vi "VBAI_MeasurementReader.vi"() -> ()   [LabVIEW 2014]
uses:
  g_Stop.vi
  g_VBAIMeasurements.vi
panel:
  in  "stop":bool
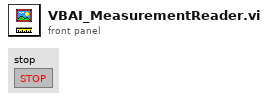
[diagram p1: front panel]
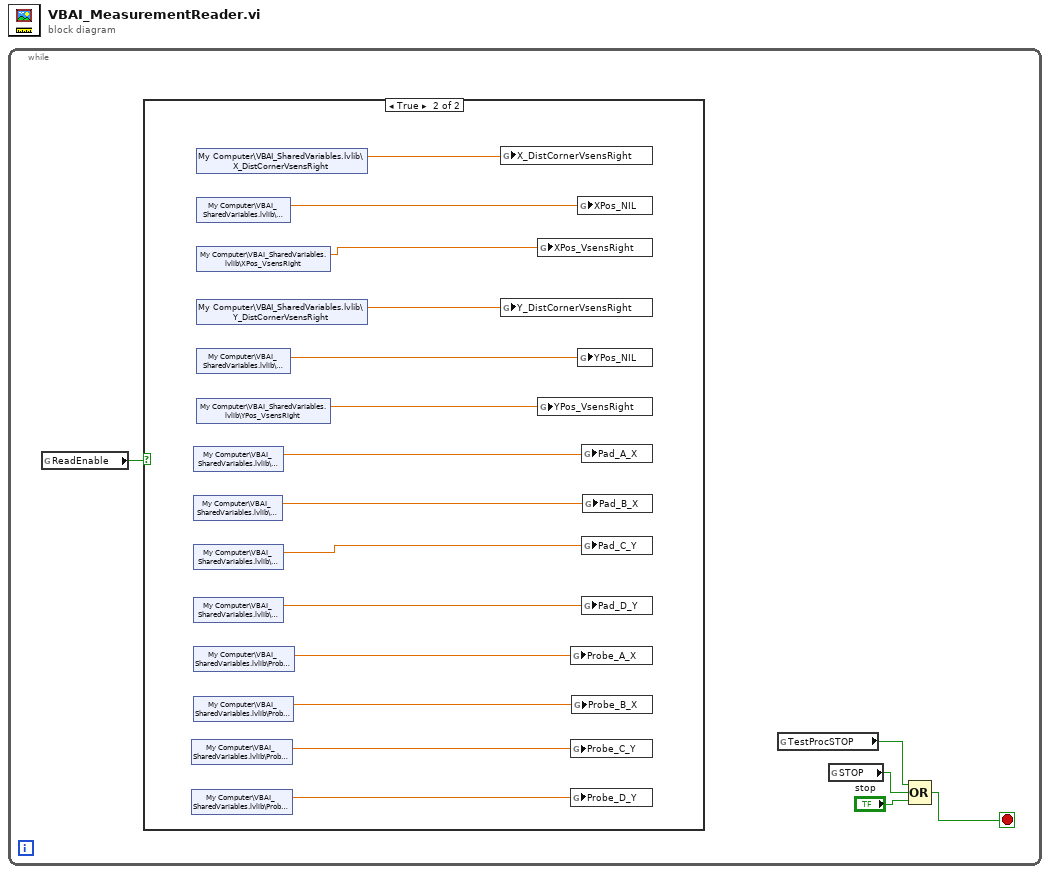
[diagram p0: block diagram]
diagram:
  n1 = while {
    stop <- w4 stop-if-true
    n2 = global read "g_VBAIMeasurements.vi" "ReadEnable"() -> (w1:bool)
    n3 = case shown="True" w1 {
      frame False {
      }
      frame True {
        n4 = shared-variable "My Computer\\VBAI_SharedVariables.lvlib\\Probe_C_Y"() -> (w7:dbl)  [unwired: 1 in, 1 out]
        n5 = shared-variable "My Computer\\VBAI_SharedVariables.lvlib\\Probe_D_Y"() -> (w6:dbl)  [unwired: 1 in, 1 out]
        n6 = shared-variable "My Computer\\VBAI_SharedVariables.lvlib\\Pad_A_X"() -> (w8:dbl)  [unwired: 1 in, 1 out]
        n7 = shared-variable "My Computer\\VBAI_SharedVariables.lvlib\\Pad_B_X"() -> (w9:dbl)  [unwired: 1 in, 1 out]
        n8 = shared-variable "My Computer\\VBAI_SharedVariables.lvlib\\Pad_C_Y"() -> (w10:dbl)  [unwired: 1 in, 1 out]
        n9 = shared-variable "My Computer\\VBAI_SharedVariables.lvlib\\Pad_D_Y"() -> (w11:dbl)  [unwired: 1 in, 1 out]
        n10 = shared-variable "My Computer\\VBAI_SharedVariables.lvlib\\Probe_A_X"() -> (w12:dbl)  [unwired: 1 in, 1 out]
        n11 = shared-variable "My Computer\\VBAI_SharedVariables.lvlib\\Probe_B_X"() -> (w13:dbl)  [unwired: 1 in, 1 out]
        n12 = shared-variable "My Computer\\VBAI_SharedVariables.lvlib\\X_DistCornerVsensRight"() -> (w19:dbl)  [unwired: 1 in, 1 out]
        n13 = shared-variable "My Computer\\VBAI_SharedVariables.lvlib\\XPos_NIL"() -> (w18:dbl)  [unwired: 1 in, 1 out]
        n14 = shared-variable "My Computer\\VBAI_SharedVariables.lvlib\\XPos_VsensRight"() -> (w17:dbl)  [unwired: 1 in, 1 out]
        n15 = shared-variable "My Computer\\VBAI_SharedVariables.lvlib\\Y_DistCornerVsensRight"() -> (w16:dbl)  [unwired: 1 in, 1 out]
        n16 = shared-variable "My Computer\\VBAI_SharedVariables.lvlib\\YPos_NIL"() -> (w15:dbl)  [unwired: 1 in, 1 out]
        n17 = shared-variable "My Computer\\VBAI_SharedVariables.lvlib\\YPos_VsensRight"() -> (w14:dbl)  [unwired: 1 in, 1 out]
        n18 = global write "g_VBAIMeasurements.vi" "X_DistCornerVsensRight"(w19) -> ()
        n19 = global write "g_VBAIMeasurements.vi" "Y_DistCornerVsensRight"(w16) -> ()
        n20 = global write "g_VBAIMeasurements.vi" "XPos_VsensRight"(w17) -> ()
        n21 = global write "g_VBAIMeasurements.vi" "YPos_VsensRight"(w14) -> ()
        n22 = global write "g_VBAIMeasurements.vi" "Probe_A_X"(w12) -> ()
        n23 = global write "g_VBAIMeasurements.vi" "Probe_C_Y"(w7) -> ()
        n24 = global write "g_VBAIMeasurements.vi" "Probe_D_Y"(w6) -> ()
        n25 = global write "g_VBAIMeasurements.vi" "Probe_B_X"(w13) -> ()
        n26 = global write "g_VBAIMeasurements.vi" "XPos_NIL"(w18) -> ()
        n27 = global write "g_VBAIMeasurements.vi" "YPos_NIL"(w15) -> ()
        n28 = global write "g_VBAIMeasurements.vi" "Pad_A_X"(w8) -> ()
        n29 = global write "g_VBAIMeasurements.vi" "Pad_C_Y"(w10) -> ()
        n30 = global write "g_VBAIMeasurements.vi" "Pad_D_Y"(w11) -> ()
        n31 = global write "g_VBAIMeasurements.vi" "Pad_B_X"(w9) -> ()
      }
    }
    n32 = global read "g_Stop.vi" "TestProcSTOP"() -> (w2:bool)
    n33 = global read "g_Stop.vi" "STOP"() -> (w3:bool)
    n34 = Compound Arithmetic op=OR(w2, w3, "stop") -> (w4:bool)
  }
